vi "CloseOtherReentrantVI.vi"(8 "error in (no error)":errorcluster, 11 "current queue name":string) -> (0 "error out":errorcluster)   [LabVIEW 2009]
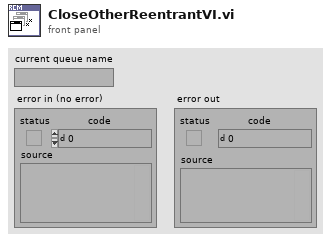
[diagram p1: front panel]
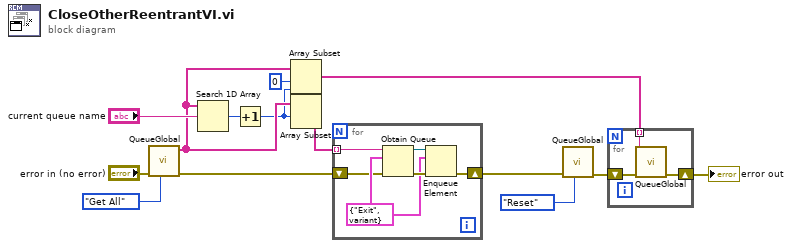
[diagram p0: block diagram]
diagram:
  n1 = call "QueueGlobal.vi"("cmd (Add)"=enum16{"Add One to End", "Get All", "Reset"}."Get All", "error in (no error)"="error in (no error)") -> ("error out"=w5:errorcluster, "queue names"=w12:string[])  [unwired: 8 in]
  n2 = Search 1D Array(1D array=w12, element="current queue name") -> (index of element=w11:i32)  [unwired: 1 in]
  n3 = Increment(x=w11) -> (x+1=w6:i32)
  n4 = Array Subset(array=w12, index=0, length=w6) -> (w7:string[])
  n5 = Array Subset(array=w12, index=w6) -> (w4:string[])  [unwired: 1 in]
  n6 = for {
    shift-right: [w20] -> w3
    shift-left: w5 -> [w15]
    tunnel: w4 -> [w16] mode=indexing
    w17 = cluster{"State":string, "Data":variant} {"State"="Exit", "Data"=variant} ("element")
    n7 = Obtain Queue(name (unnamed)=w16, element data type=w17, error in (no error)=w15) -> (queue out=w19:refnum<queue>, error out=w18:errorcluster)  [unwired: 2 in, 1 out]
    n8 = Enqueue Element(queue=w19, element=w17, error in (no error)=w18) -> (error out=w20:errorcluster)  [unwired: 1 in, 2 out]
  }
  n9 = call "QueueGlobal.vi"("cmd (Add)"=enum16{"Add One to End", "Get All", "Reset"}."Reset", "error in (no error)"=w3) -> ("error out"=w8:errorcluster)  [unwired: 8 in, 1 out]
  n10 = for {
    tunnel: w7 -> [w22] mode=indexing
    shift-right: [w21] -> w2
    shift-left: w8 -> [w23]
    n11 = call "QueueGlobal.vi"("error in (no error)"=w23, "queue name"=w22) -> ("error out"=w21:errorcluster)  [unwired: 8 in, 1 out]
  }
  "error out" <- w2
